vi "platform2Channel_Digital.vi"(9 "mazeDirection":string, 11 "Platforms":i32[](array[numeric])) -> (3 "channels":i32[](array[numeric]))   [LabVIEW 2017]
uses:
  <vilib>/imath/engines/lvmath2/RunTimeEngine/Managers/WorkSpace/UID Generator.vi
  <vilib>/imath/engines/lvmath2/RunTimeEngine/BuiltInFunctions/length/NIMS_length(GV).vi
  <instcachedir>/0/NIMS_length(GV)_08A3D13377FD4E4B96F5795FBF3698FA.lvgen/NIMS_length(GV)_08A3D13377FD4E4B96F5795FBF3698FA_002.vi
  <vilib>/imath/engines/lvmath2/RunTimeEngine/RunTimeType/NIMS_RunTimeType_From StrictType (excl LVString).vi
  <instcachedir>/0/NIMS_RunTimeType_From StrictType (excl LVString)_1019F277F0A747EDBCA0F6C52CA54500.lvgen/NIMS_RunTimeType_From StrictType (excl LVString)_1019F277F0A747EDBCA0F6C52CA54500_000.vi
  <vilib>/imath/engines/lvmath2/RunTimeEngine/LocalVariableDefStatement/MC_LocalVariableDefStatement_Display.vi
  <vilib>/imath/engines/lvmath2/RunTimeEngine/RangeToken/NIMS_Range_R2 - Integer.vi
  <instcachedir>/0/NIMS_Range_R2 - Integer_B2C3C6B11D0E4F789E1772ACB483EB02.lvgen/NIMS_Range_R2 - Integer_B2C3C6B11D0E4F789E1772ACB483EB02_000.vi
  <vilib>/imath/engines/lvmath2/RunTimeEngine/CommandStatement/MC_CommandStatement_break.vi
  <vilib>/imath/engines/lvmath2/RunTimeEngine/IndexRead/NIMS V(S).vi
  <instcachedir>/0/NIMS V(S)_0488751826AF41519A22953C041130DC.lvgen/NIMS V(S)_0488751826AF41519A22953C041130DC_002.vi
  <vilib>/imath/engines/lvmath2/RunTimeEngine/BuiltInFunctions/findnz/NIMS_[1o]_findnz(GRowV).vi
  <instcachedir>/0/NIMS_[1o]_findnz(GRowV)_3E31462E2BB14E3DAA95AD1E75EDC533.lvgen/NIMS_[1o]_findnz(GRowV)_3E31462E2BB14E3DAA95AD1E75EDC533_000.vi
  <vilib>/imath/engines/lvmath2/RunTimeEngine/IndexReplace/NIMS V(S)=V.vi
  <instcachedir>/0/NIMS V(S)=V_0F09E4CBC96B4B66B2C697D1E4CA8BB4.lvgen/NIMS V(S)=V_0F09E4CBC96B4B66B2C697D1E4CA8BB4_000.vi
  <vilib>/imath/engines/lvmath2/RunTimeEngine/ErrorHandling/NIMS_Create Error From Enums.vi
  <vilib>/imath/engines/lvmath2/RunTimeEngine/Managers/SymbolTable/Clear UID.vi
  <vilib>/imath/engines/lvmath2/RunTimeEngine/NodeEndStatement/NIMS_NodeEndStatement_Output.vi
  <instcachedir>/0/NIMS_NodeEndStatement_Output_53EC0D466D134D7ABD903AC30B43404B.lvgen/NIMS_NodeEndStatement_Output_53EC0D466D134D7ABD903AC30B43404B_005.vi
  <vilib>/imath/engines/lvmath2/RunTimeEngine/ErrorHandling/NIMS_Finalize Error.vi
  <vilib>/imath/engines/lvmath2/RunTimeEngine/Managers/SymbolTable/NIMS_WorkSpace.lvlib
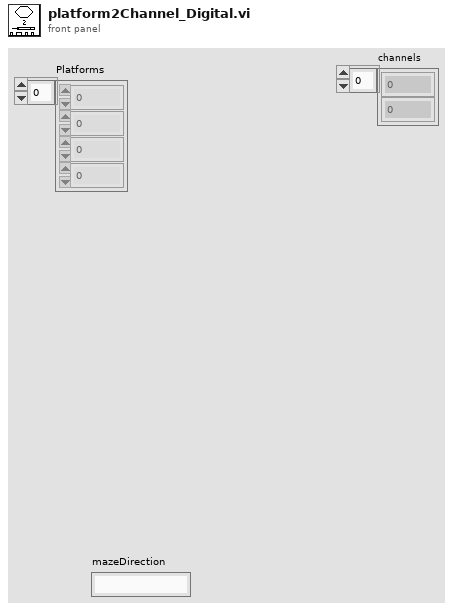
[diagram p1: front panel]
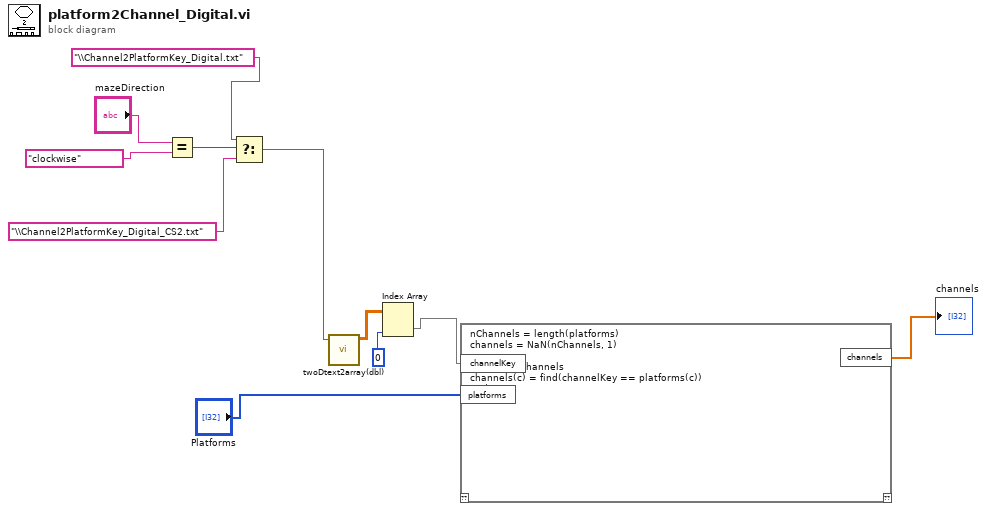
[diagram p0: block diagram]
diagram:
  n1 = Equal?(x="mazeDirection", y="clockwise") -> (x = y?=w4:bool)
  n2 = Select(t="\\Channel2PlatformKey_Digital.txt" ("String"), s=w4, f="\\Channel2PlatformKey_Digital_CS2.txt" ("String")) -> (s? t:f=w2:string)
  n3 = call "twoDtext2array(dbl).vi"("String"=w2) -> ("all rows"=w9:dbl[][])  [unwired: 10 in]
  n4 = Index Array(array=w9, index (col)=0 ("disabled index (col)")) -> (element=w7:dbl[])  [unwired: 1 in]
  n5 = mathscript code="nChannels = length(platforms)\nchannels = NaN(nChannels, 1)\n\nfor c = 1:nChannels\nchannels(c) = find(channelKey == platforms(c))\nend"("channelKey"=w7, "platforms"="Platforms") -> ("channels"=→"channels":dbl[])  [unwired: 1 in, 1 out]
